vi "GFITS_AnalizeFile.vi"(10 "line string":string, 11 "number of Extensions":u16) -> (3 "Extensions":i32[][](array[numeric]))   [LabVIEW 2016]
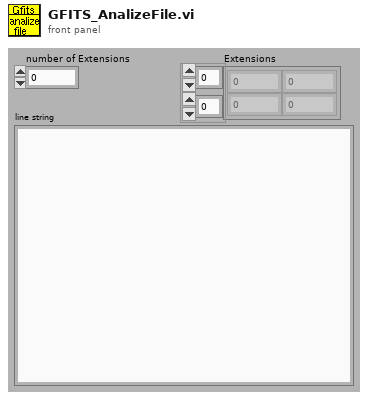
[diagram p1: front panel]
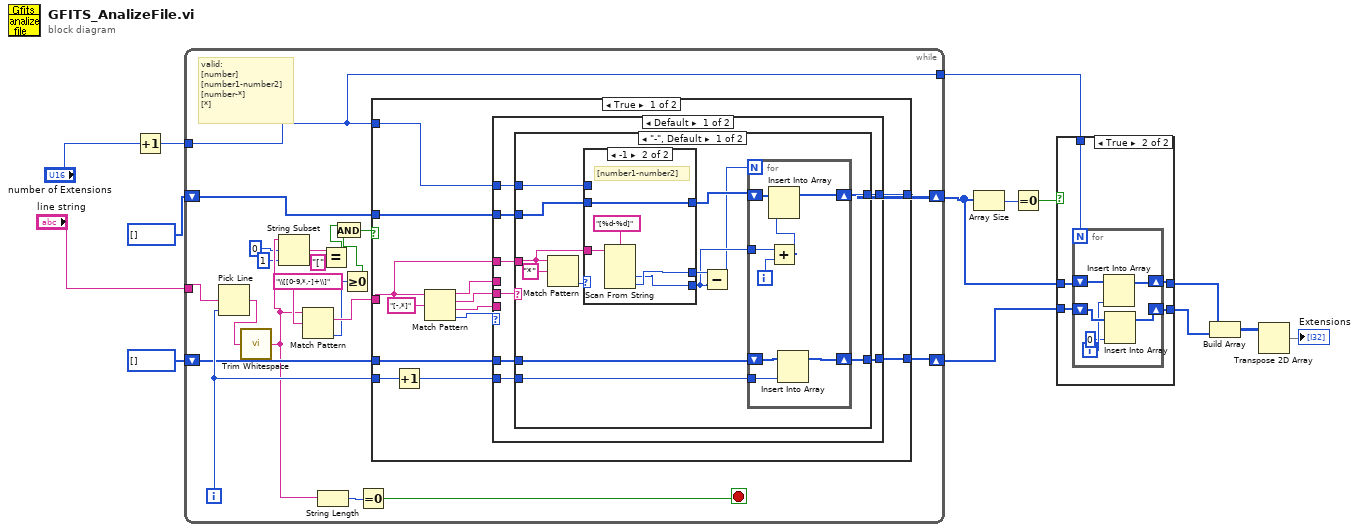
[diagram p0: block diagram]
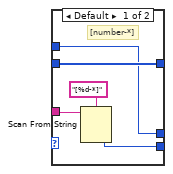
[diagram p2: hidden frame]
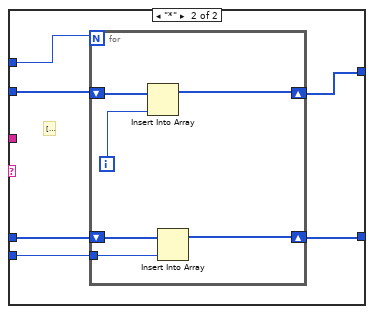
[diagram p3: hidden frame]
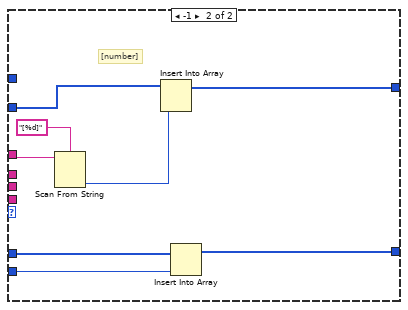
[diagram p4: hidden frame]
diagram:
  n1 = Increment(x="number of Extensions") -> (x+1=w1:u16)
  n2 = while {
    tunnel: [w25] -> w3
    shift-left: i32[] [] -> [w26]
    shift-right: [w27] -> w7
    tunnel: w1 -> [w25]
    shift-left: i32[] [] -> [w30]
    shift-right: [w31] -> w6
    tunnel: "line string" -> [w29]
    i -> [w28]
    stop <- w33 stop-if-true
    # "valid:\n[number]\n[number1-number2]\n[number-*]\n[*]"
    n3 = Pick Line(multi-line string=w29, line index=w28) -> (output string=w24:string)  [unwired: 1 out]
    n4 = call <vilib>:"Trim Whitespace.vi"("string"=w24) -> ("trimmed string"=w23:string)  [unwired: 1 in]
    n5 = String Subset(string=w23, offset (0)=0, length (rest)=1 ("length (rest)")) -> (substring=w21:string)
    n6 = Match Pattern(string=w23, regular expression="\\[[0-9,*,-]+\\]") -> (match substring=w32:string, offset past match=w19:i32)  [unwired: 3 out]
    n7 = String Length(string=w23) -> (length=w34:i32)
    n8 = Equal?(x=w21, y="[") -> (x = y?=w18:bool)
    n9 = Greater Or Equal To 0?(x=w19) -> (x >= 0?=w17:bool)
    n10 = And(x=w18, y=w17) -> (x .and. y?=w15:bool)
    n11 = Equal To 0?(x=w34) -> (x = 0?=w33:bool)
    n12 = case shown="True" w15 {
      tunnel: w32 -> [w46 _]
      tunnel: [w45 w109] -> w31
      tunnel: w30 -> [w44 w109]
      tunnel: w25 -> [w40 _]
      tunnel: w28 -> [w39 _]
      tunnel: [w38 w108] -> w27
      tunnel: w26 -> [w37 w108]
      frame True {
        n13 = Increment(x=w39) -> (x+1=w36:i32)
        n14 = Match Pattern(string=w46, regular expression="[-,*]") -> (before substring=w43:string, match substring=w41:string, after substring=w42:string, offset past match=w47:i32)  [unwired: 1 out]
        n15 = case shown="Default" w47 {
          tunnel: w46 -> [w55 w105]
          tunnel: [w52 w107] -> w45
          tunnel: w44 -> [w54 w106]
          tunnel: w43 -> [_ _]
          tunnel: w42 -> [_ _]
          tunnel: w41 -> [w56 _]
          tunnel: w40 -> [w53 _]
          tunnel: w36 -> [w50 w102]
          tunnel: [w49 w101] -> w38
          tunnel: w37 -> [w51 w100]
          frame Default {
            n16 = case shown="\"-\", Default" w56 {
              tunnel: w55 -> [w67 _]
              tunnel: w54 -> [w66 w93]
              tunnel: w53 -> [w65 w88]
              tunnel: [w61 w92] -> w52
              tunnel: w51 -> [w60 w90]
              tunnel: w50 -> [w58 w91]
              tunnel: [w59 w89] -> w49
              frame "-", Default {
                n17 = Match Pattern(string=w67, regular expression="*") -> (offset past match=w68:i32)  [unwired: 4 out]
                n18 = case shown="-1" w68 {
                  tunnel: w67 -> [w82 w86]
                  tunnel: w66 -> [w80 w83]
                  tunnel: w65 -> [w78 _]
                  tunnel: [w78 w85] -> w64
                  tunnel: [w79 w84] -> w63
                  tunnel: [w80 w83] -> w62
                  frame Default {
                    # "[number-*]"
                    n19 = Scan From String(format string="[%d-*]" ("Format String"), input string=w82) -> (output 1=w79:i32)  [unwired: 2 in, 4 out]
                  }
                  frame -1 {
                    # "[number1-number2]"
                    n20 = Scan From String(format string="[%d-%d]" ("Format String"), input string=w86) -> (output 1=w84:i32, output 2=w85:i32)  [unwired: 2 in, 5 out]
                  }
                }
                n21 = Subtract(x=w64, y=w63) -> (x-y=w57:i32)
                n22 = for {
                  N: w57 -> [_]
                  shift-right: [w75] -> w61
                  shift-left: w62 -> [w73]
                  tunnel: w63 -> [w74]
                  shift-right: [w71] -> w59
                  shift-left: w60 -> [w72]
                  tunnel: w58 -> [w70]
                  i -> [w77]
                  n23 = Add(x=w74, y=w77) -> (x+y=w76:i32)
                  n24 = Insert Into Array(array=w73, new element=w76) -> (w75:i32[])  [unwired: 1 in]
                  n25 = Insert Into Array(array=w72, new element=w70) -> (w71:i32[])  [unwired: 1 in]
                }
              }
              frame "*" {
                # "[*]"
                n26 = for {
                  N: w88 -> [_]
                  shift-right: [w94] -> w92
                  shift-left: w93 -> [w99]
                  tunnel: w91 -> [w97]
                  shift-right: [w95] -> w89
                  shift-left: w90 -> [w96]
                  i -> [w98]
                  n27 = Insert Into Array(array=w99, new element=w98) -> (w94:i32[])  [unwired: 1 in]
                  n28 = Insert Into Array(array=w96, new element=w97) -> (w95:i32[])  [unwired: 1 in]
                }
              }
            }
          }
          frame -1 {
            # "[number]"
            n29 = Scan From String(format string="[%d]" ("Format String"), input string=w105) -> (output 1=w103:i32)  [unwired: 2 in, 4 out]
            n30 = Insert Into Array(array=w106, new element=w103) -> (w107:i32[])  [unwired: 1 in]
            n31 = Insert Into Array(array=w100, new element=w102) -> (w101:i32[])  [unwired: 1 in]
          }
        }
      }
      frame False {
      }
    }
  }
  n32 = Array Size(array=w6) -> (size(s)=w9:i32)
  n33 = Equal To 0?(x=w9) -> (x = 0?=w8:bool)
  n34 = case shown="True" w8 {
    tunnel: w7 -> [w110 w115]
    tunnel: w6 -> [w111 w116]
    tunnel: [w111 w112] -> w5
    tunnel: w3 -> [_ w114]
    tunnel: [w110 w113] -> w4
    frame False {
    }
    frame True {
      n35 = for {
        N: w114 -> [_]
        shift-right: [w120] -> w112
        shift-left: w116 -> [w121]
        shift-right: [w119] -> w113
        shift-left: w115 -> [w122]
        i -> [w118]
        n36 = Insert Into Array(array=w121, new element=w118) -> (w120:i32[])  [unwired: 1 in]
        n37 = Insert Into Array(array=w122, new element=0 ("New Element/Subarray")) -> (w119:i32[])  [unwired: 1 in]
      }
    }
  }
  n38 = Build Array(w5, w4) -> (w10:i32[][])
  n39 = Transpose 2D Array(2D array=w10) -> (transposed array=→"Extensions":i32[][])
